vi "get image size.vi"(8 "error in (no error)":errorcluster, 11 "Cascade in":refnum<class "Cascade.lvclass">) -> (0 "error out":errorcluster, 3 "Cascade out":refnum<class "Cascade.lvclass">)   [LabVIEW 2012, in "Cascade.lvclass"]
uses:
  Cascade.lvclass
  Cascade.lvclass/Cascade.ctl
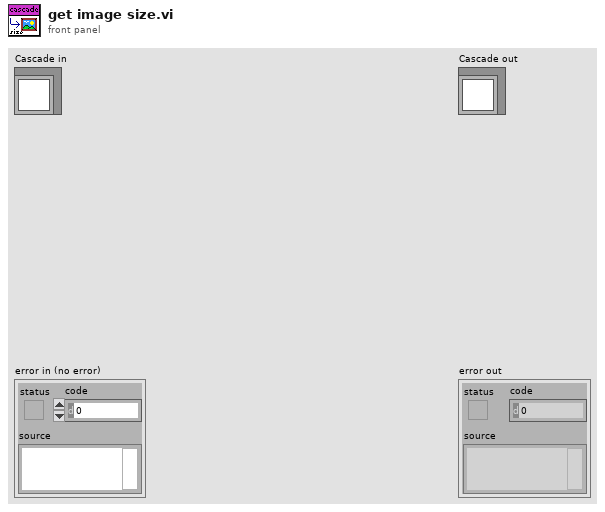
[diagram p1: front panel]
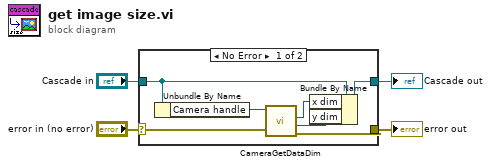
[diagram p0: block diagram]
diagram:
  n1 = case shown="No Error" "error in (no error)" {
    selector: "error in (no error)" -> [w11 w13]
    tunnel: [w10 w13] -> w3
    tunnel: [w7 w12] -> w1
    tunnel: "Cascade in" -> [w8 w12]
    frame No Error {
      n2 = Unbundle By Name(w8) -> ("Camera handle"=w9:u32)
      n3 = call <userlib>:"CameraGetDataDim.vi"("Camera Handle"=w9, "error in"=w11) -> ("Xdim"=w6:u32, "Ydim"=w5:u32, "error out"=w10:errorcluster)  [unwired: 1 out]
      n4 = Bundle By Name(cluster=w8, "x dim"=w6, "y dim"=w5) -> (w7:refnum<class "Cascade.lvclass">)
    }
    frame Error {
    }
  }
  "error out" <- w3
  "Cascade out" <- w1
